vi "read.vi"(7 "timeout (ms)":i32, 8 "error in (no error)":errorcluster, 9 "number of channels":i32, 10 "block size":i32, 11 "FPGA_AK101022Resonance in":refnum<class "FPGAWrapperAK101022Resonance.lvclass">) -> (0 "error out":errorcluster, 1 "channels raw data block":T1, 2 "FIFO full?":bool, 3 "FPGA_AK101022Resonance out":refnum<class "FPGAWrapperAK101022Resonance.lvclass">, 4 "timed out?":bool)   [LabVIEW 2010, in "FPGAWrapperAK101022Resonance.lvclass"]
uses:
  FPGAWrapperAK101022Resonance.lvclass
  common/arrays/pixel_raw_data_array.ctl
  class_data.vi
  Program Files (x86)/National Instruments/LabVIEW 2010/resource/objmgr/ni.dex.rc
panel:
  out "AvailElmntsForRead":i32
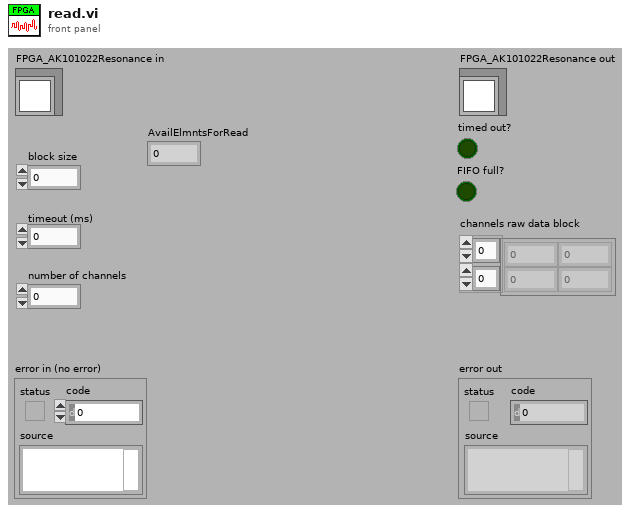
[diagram p1: front panel]
types:
  T1 = typedef "pixel_raw_data_array.ctl" = dbl[][]
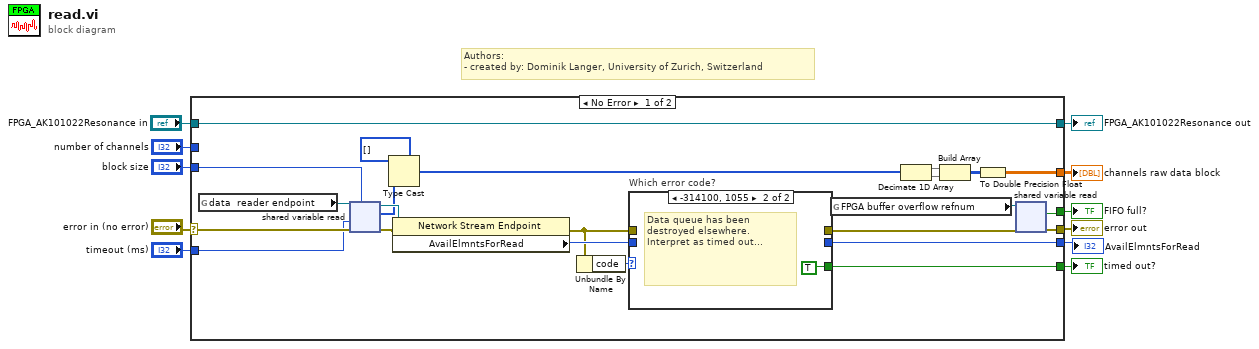
[diagram p0: block diagram]
diagram:
  # "Authors: \n- created by: Dominik Langer, University of Zurich, Switzerland"
  n1 = case shown="No Error" "error in (no error)" {
    selector: "error in (no error)" -> [w33 w39]
    tunnel: "FPGA_AK101022Resonance in" -> [w31 w38]
    tunnel: "timeout (ms)" -> [w29 _]
    tunnel: [w14 w39] -> w8
    tunnel: [w31 w38] -> w7
    tunnel: "block size" -> [w30 _]
    tunnel: "number of channels" -> [_ _]
    tunnel: [w34 _] -> w3
    tunnel: [w22 _] -> w4
    tunnel: [w13 _] -> w2
    tunnel: [w19 _] -> w1
    frame No Error {
      n2 = global read "class_data.vi" "data  reader endpoint"() -> (w32:refnum<k21>)
      n3 = shared-variable-read(w32, w33, w29, w30) -> (w18:refnum<k21>, w21:errorcluster, w12:u32[])  [unwired: 1 out]
      n4 = Type Cast(type=u16[] [], x=w12) -> (*(type *) &x=w24:u16[])
      n5 = property class="Network Stream Endpoint"(reference=w18, error in=w21) -> (error out=w17:errorcluster, "AvailElmntsForRead"=w20:i32)  [unwired: 1 out]
      n6 = Unbundle By Name(w17) -> ("code"=w23:i32)
      n7 = case "Which error code?" shown="-314100, 1055" w23 {
        tunnel: [w36 _] -> w15
        tunnel: w17 -> [w36 _]
        tunnel: [_ TRUE] -> w22
        tunnel: w20 -> [w35 _]
        tunnel: [w35 _] -> w19
        frame Default {
        }
        frame -314100, 1055 {
          # "Data queue has been destroyed elsewhere.\nInterpret as timed out..."
        }
      }
      n8 = global read "class_data.vi" "FPGA buffer overflow refnum"() -> (w16:refnum<k21>)
      n9 = Decimate 1D Array(w24) -> (w28:u16[], w27:u16[])
      n10 = Build Array(w28, w27) -> (w26:u16[][])
      n11 = To Double Precision Float(number=w26) -> (double precision float=w34:dbl[][])
      n12 = shared-variable-read(w16, w15) -> (w14:errorcluster, w13:bool)  [unwired: 2 out]
    }
    frame Error {
    }
  }
  "error out" <- w8
  "FPGA_AK101022Resonance out" <- w7
  "FIFO full?" <- w2
  "channels raw data block" <- w3
  "timed out?" <- w4
  "AvailElmntsForRead" <- w1
